vi "PS90_Disconnect.vi"(4 "error in (no error)":errorcluster, 5 "Control unit ID":i32=1 min=1 max=10, 7 "DLOwis.lvclass":refnum<class "DLOwis.lvclass">) -> (0 "error out":errorcluster, 3 "DLOwis.lvclass":refnum<class "DLOwis.lvclass">)   [LabVIEW 2018, in "DLOwis.lvclass"]
doc: "PS90_Disconnect.vi, created: 05.10.2006 alex; last change: 18.07.2016 alex;\n\n<B>FUNCTION:</B> \n\nDisconnect PS 90.\n----------------------------------------------------------------------------------------\n<B>INPUT:</B>\n[I32] <B>Control unit ID:</B> control unit index. (Default=1, Range=1...10) \n[CLU] <B>error in</B>\n----------------------------------------------------------------------------------------\n<B>OUTPUT:</B>\n[CLU] <B>error out</B>\n----------------------------------------------------------------------------------------\n<B>SUB-VIs:</B>\n----------------------------------------------------------------------------------------\n<B>EXT-Calls:</B>\nps90.dll (V2.00)\n----------------------------------------------------------------------------------------"
uses:
  DLOwis.lvclass
  C:/Dev/TRANCON/Classes/Delay Line/DelayLine.lvclass
  DelayLine.lvclass/DelayLine.ctl
  DelayLine.lvclass
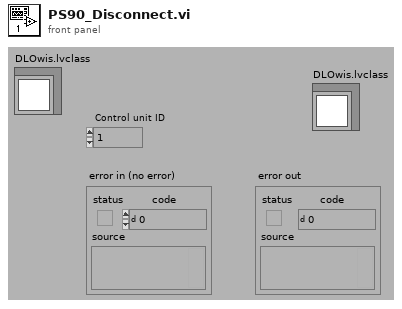
[diagram p1: front panel]
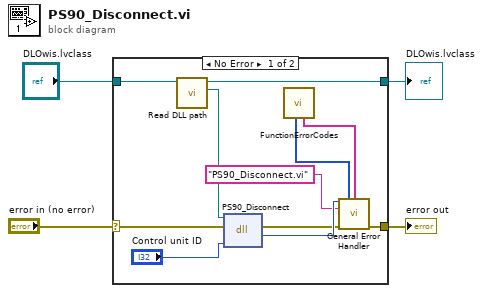
[diagram p0: block diagram]
diagram:
  n1 = case shown="No Error" "error in (no error)" {
    selector: "error in (no error)" -> [w5 w17]
    tunnel: [w14 w17] -> w4
    tunnel: [w7 w16] -> w2
    tunnel: "DLOwis.lvclass" -> [w9 w16]
    frame No Error {
      n2 = call "Read DLL path.vi"("DelayLine in"=w9) -> ("DLL path"=w8:path, "DelayLine out"=w7:refnum<class "DLOwis.lvclass">)  [unwired: 8 in, 1 out]
      n3 = dll-call lib="C:/Dev/TRANCON/DLL/ps90.dll" fn="PS90_Disconnect"(path in=w8, error in=w5, "Index"="Control unit ID") -> (error out=w6:errorcluster, "Rückgabetyp"=w13:i32)  [unwired: 2 in, 1 out]
      n4 = call "FunctionErrorCodes.vi"() -> ("[user-defined codes]"=w11:i32[], "[user-defined descriptions]"=w10:string[])  [unwired: 8 in]
      n5 = call <vilib>:"General Error Handler.vi"("[error code] (0)"=w13, "[user-defined codes]"=w11, "[user-defined descriptions]"=w10, "[error source] (\" \")"="PS90_Disconnect.vi" ("[error source] (\" \")"), "error in (no error)"=w6) -> ("error out"=w14:errorcluster)  [unwired: 6 in, 4 out]
    }
    frame Error {
    }
  }
  "error out" <- w4
  "DLOwis.lvclass" <- w2
